vi "Stop Core.vi"(10 "final error code":i32, 11 "Data Loader in":refnum<class "Data Loader.lvclass">) -> (3 "Data Loader out":refnum<class "Data Loader.lvclass">)   [LabVIEW 2020, in "Data Loader.lvlib" / "Data Loader.lvclass"]
doc: "(<B>Filename</B>: Actor Framework.lvlib:Actor.lvclass:Stop Core.vi)\n\nDefines what the actor does before it stops. Use the <B>final error code</B> input to determine whether the actor shut down in response to an error.\n\nBy default, this method passes the Stop message along to all auto-stop nested actors. A descendant class may override this method to define additional behavior, such as shutting down any processes the actor initiated in its override of the Actor Core method."
uses:
  Data Loader.lvclass
  Data Loader.lvclass/Data Loader.ctl
  MVVM Framework/MVVM Abstruct Model/MVVM Abstruct Model/MVVM Abstruct Model.lvclass
  Data Types/Abstrut Data/Abstruct Data Type.lvclass
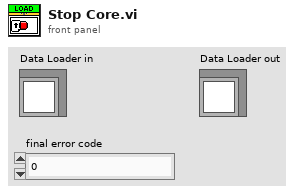
[diagram p1: front panel]
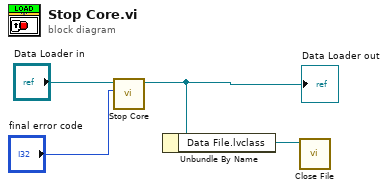
[diagram p0: block diagram]
diagram:
  n1 = call-parent "Stop Core.vi"("final error code"="final error code", "Actor in"="Data Loader in") -> ("Actor out"=w2:refnum<class "Data Loader.lvclass">)  [unwired: 9 in]
  "Data Loader out" <- w2
  n2 = Unbundle By Name(w2) -> ("Data File.lvclass"=w1:refnum<class "Abstruct Data Type.lvclass">)
  n3 = call-dynamic "Close File.vi"("Abstruct Data Type in"=w1) -> ()  [unwired: 9 in, 2 out]
